vi "Is Default.vi"(8 "error in (no error)":errorcluster, 11 "Proto Tag in":refnum<class "Basic Type.lvclass">) -> (0 "error out":errorcluster, 2 "Is Default Value?":bool, 3 "Proto Tag out":refnum<class "Basic Type.lvclass">)   [LabVIEW 2020, in "Protobuf RAW.lvlib" / "Basic Type.lvclass"]
uses:
  Basic Type.lvclass
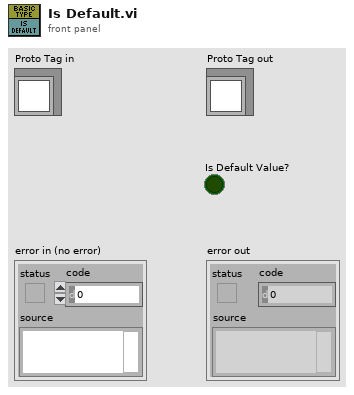
[diagram p1: front panel]
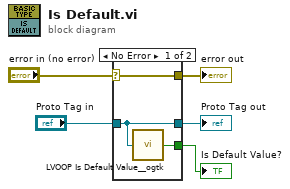
[diagram p0: block diagram]
diagram:
  n1 = case shown="No Error" "error in (no error)" {
    selector: "error in (no error)" -> [w8 w10]
    tunnel: [w8 w10] -> w4
    tunnel: [w7 w9] -> w2
    tunnel: "Proto Tag in" -> [w7 w9]
    tunnel: [w6 _] -> w1
    frame No Error {
      n2 = call <userlib>:"LVOOP Is Default Value__ogtk.vi"("Object"=w7) -> ("Is Default Value?"=w6:bool)
    }
    frame Error {
    }
  }
  "error out" <- w4
  "Proto Tag out" <- w2
  "Is Default Value?" <- w1
